vi "BACKTOBASE.vi"   [LabVIEW 2016, in "Test2.lvrbt"]
uses:
  Test2.lvrbt
  <vilib>/NXT/Subs/ColorSensorColors.ctl
  <vilib>/NXT/Block Support/NXT_InputPort.ctl
  <vilib>/NXT/Hardware/Plugins/Tetrix DC Motor/TetrixDCMotorAddress.ctl
  <vilib>/NXT/Hardware/Plugins/Tetrix 180 deg Servo/Tetrix180ServoAddress.ctl
  <vilib>/NXT/NXTIO Xnodes/NXTIONodeSubVIs/TETRIX IO Move Servos.vi
  <vilib>/NXT/Dual Mode Library/Waits/Wait_Num.vi
  <vilib>/NXT/NXTIO Xnodes/NXTIONodeSubVIs/TETRIX IO Move DC Motors.vi
  <vilib>/NXT/Dual Mode Library/Waits/Wait_EV3_Color_Color.vi
  <vilib>/NXT/NXTIO Xnodes/NXTIONodeSubVIs/TETRIX IO Stop DC Motors.vi
  <vilib>/NXT/Dual Mode Library/Waits/Wait_EV3_Ultrasonic_Centimeters_Further.vi
  <vilib>/NXT/NXTIO Xnodes/AddressXNode/NXTIOAddress.xnode
  <vilib>/NXT/Subs/LVHSConnector.ctl
  <vilib>/NXT/NXTIO Xnodes/NXTIOXNode/NXTIO.xnode
  <vilib>/NXT/LegoClasses/BrickReference/BrickReference.lvclass
types:
  T1 = typedef "NXT_InputPort.ctl" = u32
  T2 = typedef "ColorSensorColors.ctl" = enum16{"No Color", "Black", "Blue", "Green", "Yellow", "Red", "White", "Brown"}
  T3 = typedef "Tetrix180ServoAddress.ctl" = i32
  T4 = cluster{"Tetrix180Servo":T3, "Tetrix180Servo":T3, "Tetrix180Servo":T3, "Tetrix180Servo":T3, "Tetrix180Servo":T3, "Tetrix180Servo":T3}
  T5 = typedef "LVHSConnector.ctl" = refnum<class "BrickReference.lvclass">
  T6 = typedef "TetrixDCMotorAddress.ctl" = i32
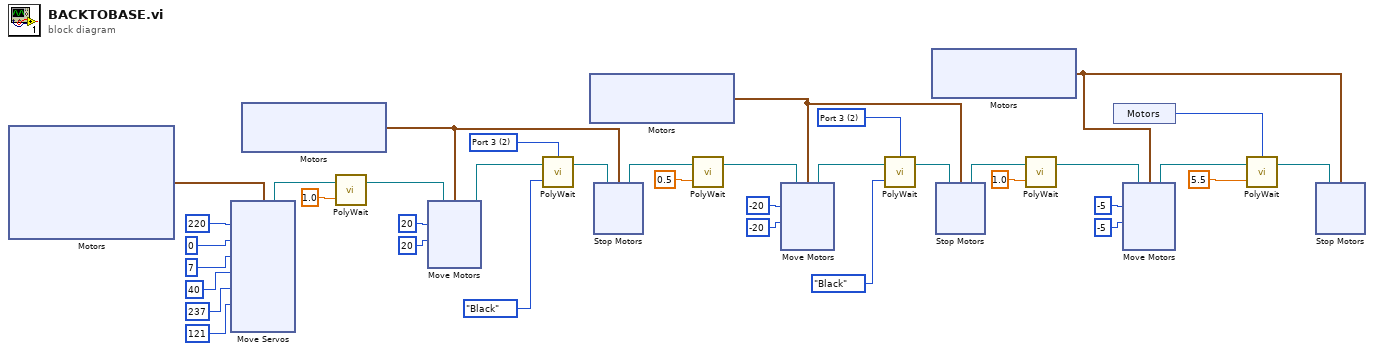
[diagram p0: block diagram]
diagram:
  w22 = T1 2 items=["Port 1", "Port 2", "Port 3", "Port 4"] ("Port (Port 1)")
  w31 = T1 2 items=["Port 1", "Port 2", "Port 3", "Port 4"] ("Port (Port 1)")
  n1 = xnode "Motors"() -> ("Motor"=w20:T4)
  n2 = xnode "Move Servos"("Position 6"=u8 121, "Position 5"=u8 237, "Position 4"=u8 40, "Position 3"=u8 7, "Position 2"=u8 0, "Position 1"=u8 220, "Motors"=w20) -> ("NXT/EV3"=w12:T5)  [unwired: 1 in]
  n3 = xnode "Motors"() -> ("Motor"=w33:cluster{"TetrixDCMotor":T6, "TetrixDCMotor":T6})
  n4 = call-poly <vilib>:"PolyWait.vi"("Time (1 sec)"=sgl 1.0, "NXT/EV3"=w12) -> ("NXT/EV3"=w11:T5)  [unwired: 2 in]
  n5 = xnode "Move Motors"("Power/Speed 2"=i8 20, "Power/Speed 1"=i8 20, "Motors"=w33, "NXT/EV3"=w11) -> ("NXT/EV3"=w35:T5)
  n6 = call-poly <vilib>:"PolyWait.vi"("Color (Red)"=ColorSensorColors."Black", "NXT/EV3"=w35, "Port (Port 1)"=w31) -> ("NXT/EV3"=w34:T5)  [unwired: 1 in]
  n7 = xnode "Motors"() -> ("Motor"=w26:cluster{"TetrixDCMotor":T6, "TetrixDCMotor":T6})
  n8 = xnode "Stop Motors"("Motors"=w33, "NXT/EV3"=w34) -> ("NXT/EV3"=w21:T5)
  n9 = call-poly <vilib>:"PolyWait.vi"("Time (1 sec)"=sgl 0.5, "NXT/EV3"=w21) -> ("NXT/EV3"=w24:T5)  [unwired: 2 in]
  n10 = xnode "Move Motors"("Power/Speed 2"=i8 -20, "Power/Speed 1"=i8 -20, "Motors"=w26, "NXT/EV3"=w24) -> ("NXT/EV3"=w28:T5)
  n11 = call-poly <vilib>:"PolyWait.vi"("Color (Red)"=ColorSensorColors."Black", "NXT/EV3"=w28, "Port (Port 1)"=w22) -> ("NXT/EV3"=w27:T5)  [unwired: 1 in]
  n12 = xnode "Motors"() -> ("Motor"=w5:cluster{"TetrixDCMotor":T6, "TetrixDCMotor":T6})
  n13 = xnode "Stop Motors"("Motors"=w26, "NXT/EV3"=w27) -> ("NXT/EV3"=w3:T5)
  n14 = call-poly <vilib>:"PolyWait.vi"("Time (1 sec)"=sgl 1.0, "NXT/EV3"=w3) -> ("NXT/EV3"=w2:T5)  [unwired: 2 in]
  n15 = xnode "Motors"() -> ("Sensor"=w1:T1)
  n16 = xnode "Move Motors"("Power/Speed 2"=i8 -5, "Power/Speed 1"=i8 -5, "Motors"=w5, "NXT/EV3"=w2) -> ("NXT/EV3"=w8:T5)
  n17 = call-poly <vilib>:"PolyWait.vi"("Centimeters (50)"=sgl 5.5 ("Time (1 sec)"), "NXT/EV3"=w8, "Port (Port 1)"=w1) -> ("NXT/EV3"=w6:T5)  [unwired: 1 in]
  n18 = xnode "Stop Motors"("Motors"=w5, "NXT/EV3"=w6) -> ()  [unwired: 1 out]
